vi "CreateMethodTree.vi"(6 "DisabledMethodsNames":T1(array[cluster]), 8 "error in (no error)":errorcluster, 9 "StartSelectedMethodsPerInterfaces":T1(array[cluster]), 10 "InterfacePath":T2[](array[typedef]), 11 "TreeControlRef":refnum<vi>) -> (0 "error out":errorcluster, 1 "InterfacesTag":string[](array[string]), 2 "MethodsTagPerInterfaces":cluster{"Array":string[]}[](array[cluster]), 3 "MethodsSelectedPerInterface":cluster{"Array":bool[]}[](array[cluster]), 4 "MethodsDisabledPerInterface":cluster{"Array":bool[]}[](array[cluster]))   [LabVIEW 2020, in "InterfaceLibrary.lvlib"]
uses:
  <resource>/Framework/Providers/Open_GDS/ClassProviders/Common/InterfaceLibrary/InterfaceLibrary.lvlib
  <resource>/Framework/Providers/Open_GDS/ClassProviders/Common/InterfaceLibrary/InterfaceInfo.ctl
  <resource>/Framework/Providers/Open_GDS/ClassProviders/Common/LvClass_class/GDSLvClass_ClassMethodInfo.ctl
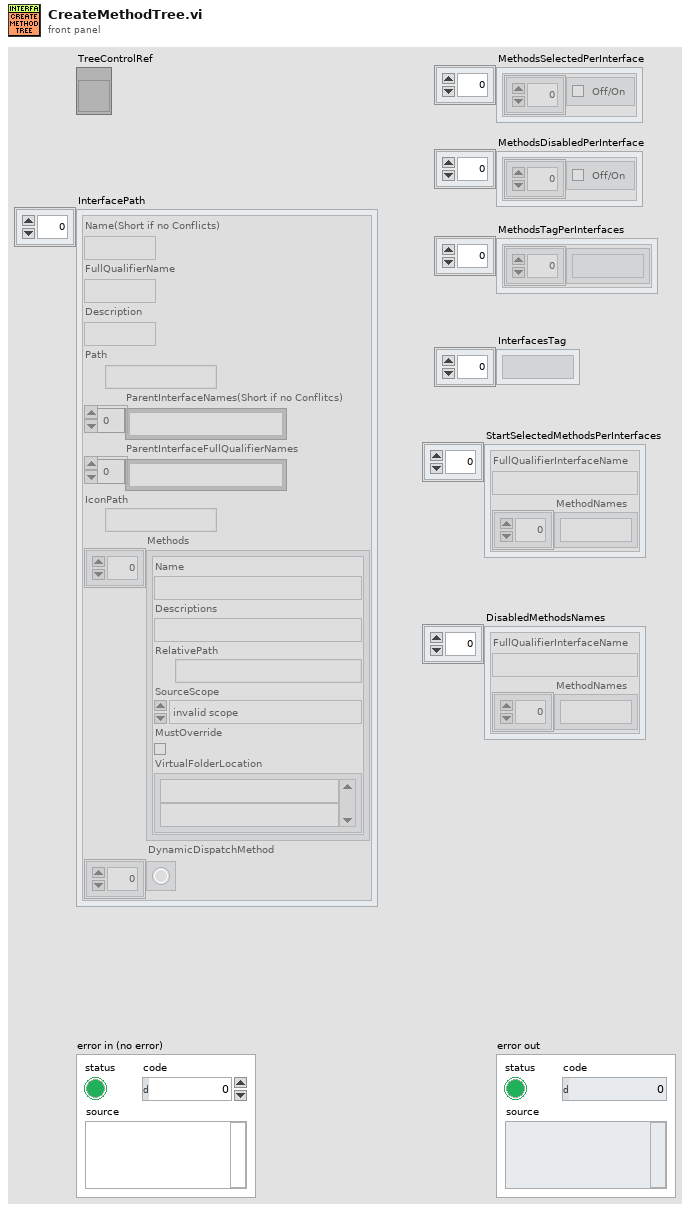
[diagram p1: front panel]
types:
  T1 = cluster{"FullQualifierInterfaceName":string, "MethodNames":string[]}[]
  T2 = typedef "InterfaceLibrary.lvlib/InterfaceInfo.ctl" = cluster{"Name(Short if no Conflicts)":string, "FullQualifierName":string, "Description":string, "Path":path, "ParentInterfaceNames(Short if no Conflitcs)":string[], "ParentInterfaceFullQualifierNames":string[], "IconPath":path, "Methods":T3[], "DynamicDispatchMethod":bool[]}
  T3 = typedef "GDSLvClass_ClassMethodInfo.ctl" = cluster{"Name":string, "Descriptions":string, "RelativePath":path, "SourceScope":enum32{"invalid scope", "public", "private", "protected", "community"}, "MustOverride":bool, "VirtualFolderLocation":string[]}
  T4 = cluster{"FullQualifierInterfaceName":string, "MethodNames":string[]}
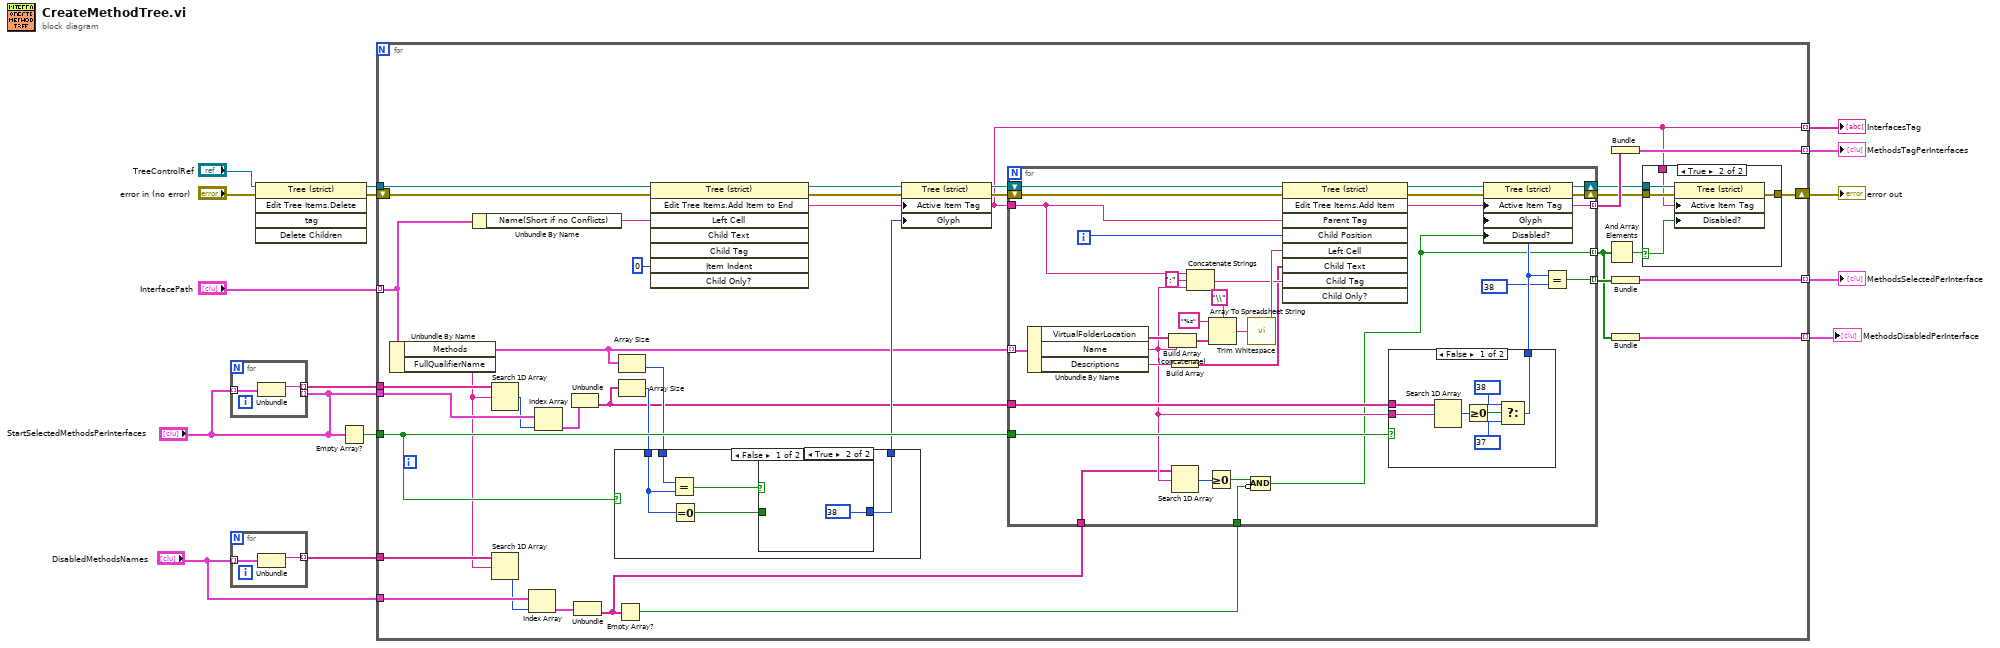
[diagram p0: block diagram]
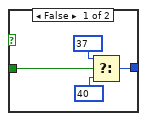
[diagram p3: hidden frame]
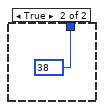
[diagram p4: hidden frame]
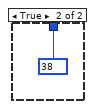
[diagram p5: hidden frame]
diagram:
  n1 = for {
    tunnel: "StartSelectedMethodsPerInterfaces" -> [w17] mode=indexing
    tunnel: [w16] -> w5 mode=indexing
    tunnel: "StartSelectedMethodsPerInterfaces" -> [_] mode=indexing
    n2 = Unbundle(w17) -> ("FullQualifierInterfaceName"=w16:string)  [unwired: 1 out]
  }
  n3 = for {
    tunnel: "DisabledMethodsNames" -> [w19] mode=indexing
    tunnel: [w18] -> w3 mode=indexing
    n4 = Unbundle(w19) -> ("FullQualifierInterfaceName"=w18:string)  [unwired: 1 out]
  }
  n5 = invoke on="Invoke Node" class="Tree (strict)" method="Edit Tree Items.Delete"(reference="TreeControlRef", error in="error in (no error)") -> (reference out=w14:refnum<vi>, error out=w7:errorcluster)  [unwired: 3 in, 3 out]
  n6 = Empty Array?(array="StartSelectedMethodsPerInterfaces") -> (empty?=w6:bool)
  n7 = for {
    tunnel: "InterfacePath" -> [w54] mode=indexing
    shift-right: [w24] -> w9
    shift-left: w7 -> [w51]
    tunnel: [w49] -> w11 mode=indexing
    tunnel: [w22] -> w10 mode=indexing
    tunnel: [w48] -> w12 mode=indexing
    tunnel: w14 -> [w47]
    tunnel: w6 -> [w44]
    tunnel: w5 -> [w39]
    tunnel: "StartSelectedMethodsPerInterfaces" -> [w38]
    tunnel: w3 -> [w34]
    tunnel: "DisabledMethodsNames" -> [w32]
    tunnel: [w20] -> w1 mode=indexing
    n8 = Unbundle By Name(w54) -> ("Methods"=w42:T3[], "FullQualifierName"=w33:string)
    n9 = Unbundle By Name(w54) -> ("Name(Short if no Conflicts)"=w56:string)
    n10 = Search 1D Array(1D array=w39, element=w33) -> (index of element=w37:i32)  [unwired: 1 in]
    n11 = Search 1D Array(1D array=w34, element=w33) -> (index of element=w31:i32)  [unwired: 1 in]
    n12 = Index Array(array=w32, index=w31) -> (element=w30:T4)
    n13 = Index Array(array=w38, index=w37) -> (element=w36:T4)
    n14 = Unbundle(w36) -> ("MethodNames"=w35:string[])  [unwired: 1 out]
    n15 = Unbundle(w30) -> ("MethodNames"=w29:string[])  [unwired: 1 out]
    n16 = Empty Array?(array=w29) -> (empty?=w28:bool)
    n17 = Array Size(array=w42) -> (size(s)=w41:i32)
    n18 = Array Size(array=w35) -> (size(s)=w40:i32)
    n19 = case shown="False" w44 {
      tunnel: [w63 38] -> w43
      tunnel: w41 -> [w67 _]
      tunnel: w40 -> [w65 _]
      frame False {
        n20 = Equal?(x=w67, y=w65) -> (x = y?=w66:bool)
        n21 = Equal To 0?(x=w65) -> (x = 0?=w64:bool)
        n22 = case shown="True" w66 {
          tunnel: w64 -> [w69 _]
          tunnel: [w68 38] -> w63
          frame False {
            n23 = Select(t=37, s=w69, f=40) -> (s? t:f=w68:i32)
          }
          frame True {
          }
        }
      }
      frame True {
      }
    }
    n24 = invoke on="Invoke Node" class="Tree (strict)" method="Edit Tree Items.Add Item to End"(reference=w47, error in=w51, "Left Cell"=w56, "Item Indent"=0 ("New Item Indentation")) -> (reference out=w46:refnum<vi>, error out=w53:errorcluster, "Edit Tree Items:Add Item to End"=w22:string)  [unwired: 4 in, 5 out]
    n25 = property on="Property Node" class="Tree (strict)"(reference=w46, error in=w53, "Active Item Tag"=w22, "Glyph"=w43) -> (reference out=w45:refnum<vi>, error out=w52:errorcluster)
    n26 = for {
      tunnel: w42 -> [w104] mode=indexing
      tunnel: w22 -> [w93]
      shift-right: [w94] -> w25
      shift-left: w52 -> [w98]
      tunnel: [w84] -> w50 mode=indexing
      tunnel: w44 -> [w86]
      tunnel: w35 -> [w85]
      tunnel: w29 -> [w82]
      tunnel: w28 -> [w79]
      tunnel: [w76] -> w27 mode=indexing
      tunnel: [w75] -> w21 mode=indexing
      shift-right: [w74] -> w23
      shift-left: w45 -> [w88]
      i -> [w97]
      n27 = Unbundle By Name(w104) -> ("VirtualFolderLocation"=w103:string[], "Name"=w83:string, "Descriptions"=w90:string)
      n28 = Build Array (concatenate)(w103, w83) -> (w102:string[])
      n29 = Build Array(w90) -> (w89:string[])
      n30 = Search 1D Array(1D array=w82, element=w83) -> (index of element=w81:i32)  [unwired: 1 in]
      n31 = Concatenate Strings(w93, ":" ("string"), w83) -> (w92:string)
      n32 = Greater Or Equal To 0?(x=w81) -> (x >= 0?=w80:bool)
      n33 = Array To Spreadsheet String(delimiter (Tab)="\\", array=w102, 3:"%s" ("format string")) -> (spreadsheet string=w99:string)
      n34 = call <vilib>:"Trim Whitespace.vi"("string"=w99) -> ("trimmed string"=w96:string)  [unwired: 1 in]
      n35 = Compound Arithmetic op=AND(w80, invert w79) -> (w75:bool)
      n36 = invoke on="Invoke Node" class="Tree (strict)" method="Edit Tree Items.Add Item"(reference=w88, error in=w98, "Parent Tag"=w93, "Child Position"=w97, "Left Cell"=w96, "Child Text"=w89, "Child Tag"=w92) -> (reference out=w87:refnum<vi>, error out=w95:errorcluster, "Edit Tree Items:Add Item"=w84:string)  [unwired: 2 in, 6 out]
      n37 = case shown="False" w86 {
        tunnel: [w105 38] -> w78
        tunnel: w85 -> [w111 _]
        tunnel: w83 -> [w110 _]
        frame False {
          n38 = Search 1D Array(1D array=w111, element=w110) -> (index of element=w109:i32)  [unwired: 1 in]
          n39 = Greater Or Equal To 0?(x=w109) -> (x >= 0?=w108:bool)
          n40 = Select(t=38, s=w108, f=37) -> (s? t:f=w105:i32)
        }
        frame True {
        }
      }
      n41 = property on="Property Node" class="Tree (strict)"(reference=w87, error in=w95, "Active Item Tag"=w84, "Glyph"=w78, "Disabled?"=w75) -> (reference out=w74:refnum<vi>, error out=w94:errorcluster)
      n42 = Equal?(x=w78, y=38) -> (x = y?=w76:bool)
    }
    n43 = And Array Elements(Boolean array=w21) -> (logical AND=w26:bool)
    n44 = Bundle(w50) -> (w49:cluster{string[]})  [unwired: 1 in]
    n45 = Bundle(w27) -> (w48:cluster{bool[]})  [unwired: 1 in]
    n46 = Bundle(w21) -> (w20:cluster{bool[]})  [unwired: 1 in]
    n47 = case shown="True" w26 {
      selector: w26 -> [_ w58]
      tunnel: w25 -> [w57 w62]
      tunnel: [w57 w61] -> w24
      tunnel: w23 -> [_ w60]
      tunnel: w22 -> [_ w59]
      frame False {
      }
      frame True {
        n48 = property on="Property Node" class="Tree (strict)"(reference=w60, error in=w62, "Active Item Tag"=w59, "Disabled?"=w58) -> (error out=w61:errorcluster)  [unwired: 1 out]
      }
    }
  }
  "MethodsSelectedPerInterface" <- w12
  "MethodsTagPerInterfaces" <- w11
  "InterfacesTag" <- w10
  "error out" <- w9
  "MethodsDisabledPerInterface" <- w1
